vi "StandAloneApp.vi"() -> ()   [LabVIEW 2016]
uses:
  VIs/ColorText/Code.xctl
panel:
  in  "Tab Control":enum32{"IntroPage", "Choose"}(tab)
  in  "MoveOn":bool
  in  "Run":bool
  out "Code":string(xcontrol)
  in  "Backpack?":bool
  in  "Spike?":bool
  in  "Templates":i32(listbox)
  in  "Spike Name":string="Select"
  in  "Backpack":string="Select"
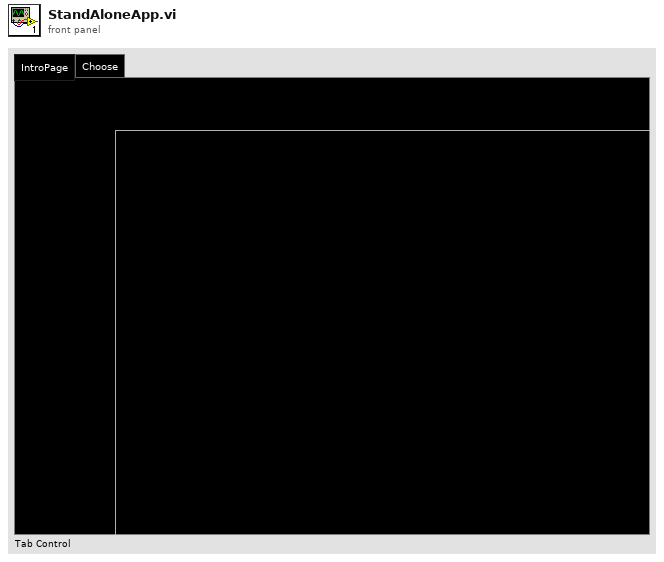
[diagram p1: front panel]
types:
  T1 = enum8{"Enabled", "Disabled", "Disabled and Grayed Out"}
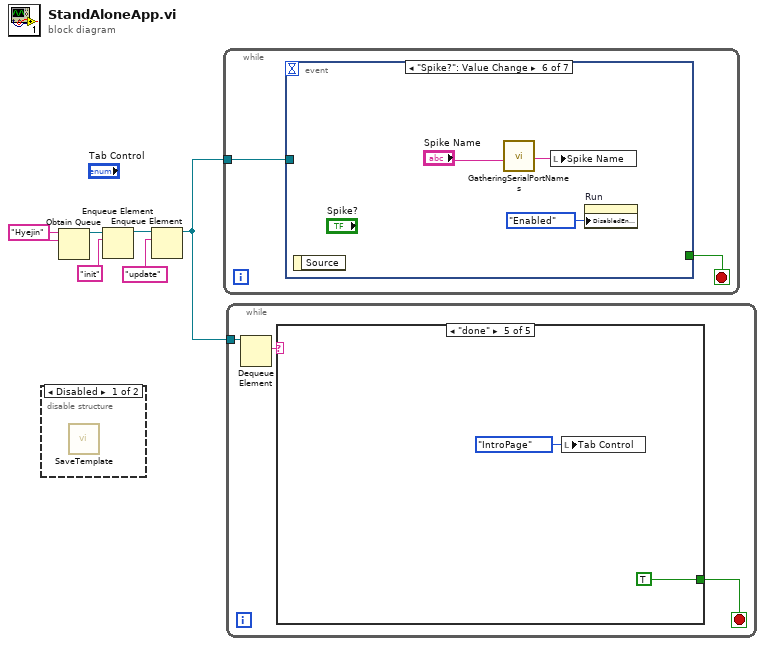
[diagram p0: block diagram]
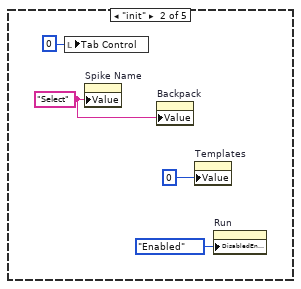
[diagram p4: hidden frame]
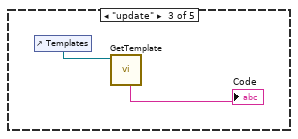
[diagram p5: hidden frame]
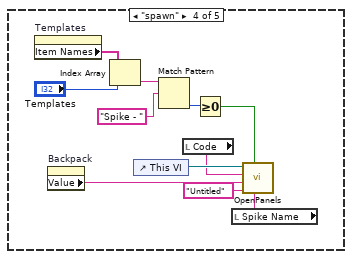
[diagram p6: hidden frame]
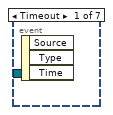
[diagram p7: hidden frame]
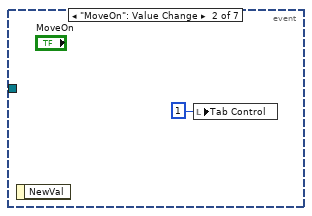
[diagram p8: hidden frame]
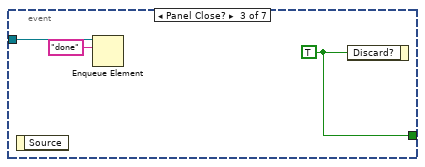
[diagram p9: hidden frame]
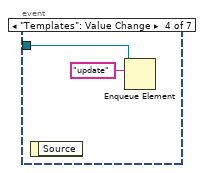
[diagram p10: hidden frame]
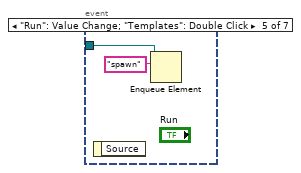
[diagram p11: hidden frame]
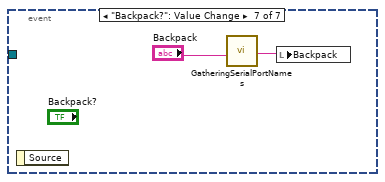
[diagram p12: hidden frame]
diagram:
  w4 = "Hyejin" ("name (unnamed)")
  n1 = disable-structure shown="Disabled" {
    frame Disabled {
      n2 = call "SaveTemplate.vi"() -> ()  [unwired: 12 in]
    }
    frame Enabled {
    }
  }
  n3 = Obtain Queue(name (unnamed)=w4, element data type=w4) -> (queue out=w6:refnum<queue>)  [unwired: 3 in, 2 out]
  n4 = Enqueue Element(queue=w6, element="init") -> (queue out=w3:refnum<queue>)  [unwired: 2 in, 2 out]
  n5 = Enqueue Element(queue=w3, element="update") -> (queue out=w2:refnum<queue>)  [unwired: 2 in, 2 out]
  n6 = while {
    tunnel: w2 -> [w7]
    stop <- w8 stop-if-true
    n7 = event shown="[5] \"Spike?\": Value Change" {
      selector: _ -> [_ _ _ _ _ _ _]
      dyn-events: _ -> [_ _ _ _ _ _ _]
      timeout: _ -> [_ _ _ _ _ _ _]
      tunnel: [_ _ w12 _ _ _ _] -> w8
      tunnel: w7 -> [_ _ w10 w13 w15 _ _]
      event Timeout {
        n8 = event-data() -> ()  [unwired: 1 in, 3 out]
      }
      event "MoveOn": Value Change {
        n9 = event-data() -> ()  [unwired: 1 in, 1 out]
        n10 = local write "Tab Control"(1) -> ()
      }
      event Panel Close? {
        w12 = TRUE ("Discard?")
        n11 = event-data() -> ()  [unwired: 1 in, 1 out]
        n12 = Enqueue Element(queue=w10, element="done") -> ()  [unwired: 2 in, 3 out]
        n13 = event-data("Discard?"=w12) -> ()  [unwired: 1 in, 1 out]
      }
      event "Templates": Value Change {
        n14 = event-data() -> ()  [unwired: 1 in, 1 out]
        n15 = Enqueue Element(queue=w13, element="update") -> ()  [unwired: 2 in, 3 out]
      }
      event "Run": Value Change; "Templates": Double Click {
        n16 = event-data() -> ()  [unwired: 1 in, 1 out]
        n17 = Enqueue Element(queue=w15, element="spawn") -> ()  [unwired: 2 in, 3 out]
      }
      event "Spike?": Value Change {
        n18 = event-data() -> ()  [unwired: 1 in, 1 out]
        n19 = call "GatheringSerialPortNames.vi"("old Name"="Spike Name") -> ("name"=w18:string)  [unwired: 10 in]
        n20 = local write "Spike Name"(w18) -> ()
        n21 = property on="Run" class="Bool"("DisabledEnum"=T1."Enabled" ("Disabled")) -> ()  [unwired: 2 in, 2 out]
      }
      event "Backpack?": Value Change {
        n22 = event-data() -> ()  [unwired: 1 in, 1 out]
        n23 = call "GatheringSerialPortNames.vi"("old Name"="Backpack") -> ("name"=w20:string)  [unwired: 10 in]
        n24 = local write "Backpack"(w20) -> ()
      }
    }
  }
  n25 = while {
    tunnel: w2 -> [w23]
    stop <- w22 stop-if-true
    n26 = Dequeue Element(queue=w23) -> (element=w24:string)  [unwired: 2 in, 3 out]
    n27 = case shown="\"done\"" w24 {
      tunnel: [_ _ _ _ TRUE ("Discard?")] -> w22
      frame Default {
      }
      frame "init" {
        w27 = "Select" ("Value")
        n28 = local write "Tab Control"(0) -> ()
        n29 = property on="Spike Name" class="Str"("Value"=w27) -> ()  [unwired: 2 in, 2 out]
        n30 = property on="Backpack" class="Str"("Value"=w27) -> ()  [unwired: 2 in, 2 out]
        n31 = property on="Templates" class="LstBox (strict)"("Value"=0 ("Value (Signaling)")) -> ()  [unwired: 2 in, 2 out]
        n32 = property on="Run" class="Bool"("DisabledEnum"=T1."Enabled" ("Disabled")) -> ()  [unwired: 2 in, 2 out]
      }
      frame "update" {
        n33 = control-ref of="Templates"() -> (w30:refnum<vi>)
        n34 = call "GetTemplate.vi"("ListBox in"=w30) -> ("Python"=→"Code":string)  [unwired: 10 in]
      }
      frame "spawn" {
        n35 = property on="Templates" class="LstBox (strict)"() -> ("Item Names"=w36:string[])  [unwired: 2 in, 2 out]
        n36 = property on="Backpack" class="Str"() -> ("Value"=w38:string)  [unwired: 2 in, 2 out]
        n37 = Index Array(array=w36, index="Templates") -> (element=w32:string)
        n38 = control-ref of="This VI"() -> (w41:refnum<vi>)
        n39 = Match Pattern(string=w32, regular expression="Spike - ") -> (offset past match=w34:i32)  [unwired: 1 in, 3 out]
        n40 = local read "Code"() -> (w40:string)
        n41 = Greater Or Equal To 0?(x=w34) -> (x >= 0?=w31:bool)
        n42 = local read "Spike Name"() -> (w39:string)
        n43 = call "OpenPanels.vi"("Spike"=w39, "Single?"=w31, "File Name"="Untitled", "Backpack"=w38, "Code"=w40, "VI in"=w41) -> ()  [unwired: 6 in]
      }
      frame "done" {
        n44 = local write "Tab Control"(enum32{"IntroPage", "Choose"}."IntroPage" ("Tab Control")) -> ()
      }
    }
  }
